vi "test Start Clear.vi"(8 "error in (no error)":errorcluster, 11 "TestCase in":refnum<class "Channel Manager.lvclass">) -> (0 "error out":errorcluster, 3 "TestCase out":refnum<class "Channel Manager.lvclass">)   [LabVIEW 2020, in "Channel Manager.lvclass"]
uses:
  Channel Manager.lvclass
  Hardware API/Channel Status.ctl
  Hardware API/Channel Action.ctl
  <vilib>/addons/_JKI Toolkits/VI Tester/TestCase.llb/TestCase.lvclass
  Hardware API/AIM ARINC 429 Hardware API.lvlib
  C:/Program Files (x86)/National Instruments/LabVIEW 2020/vi.lib/addons/_JKI Toolkits/VI Tester/TestCase.llb/TestCase.lvclass
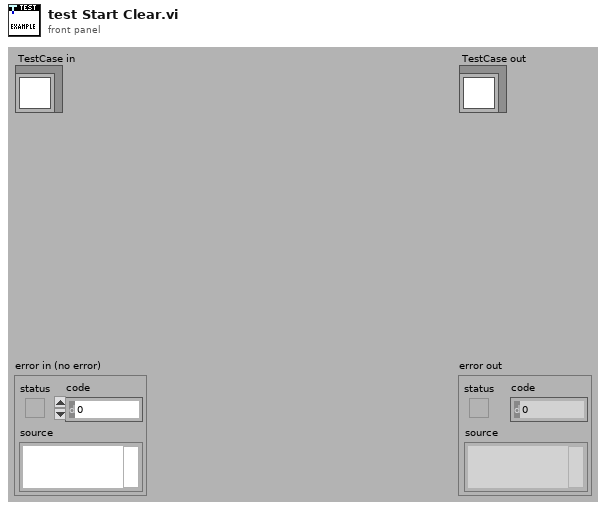
[diagram p1: front panel]
types:
  T1 = typedef "AIM ARINC 429 Hardware API.lvlib/Channel Status.ctl" = enum16{"Uninitialized", "Idle", "Active"}
  T2 = typedef "AIM ARINC 429 Hardware API.lvlib/Channel Action.ctl" = enum16{"Get Info", "Initialize", "Start", "Clear"}
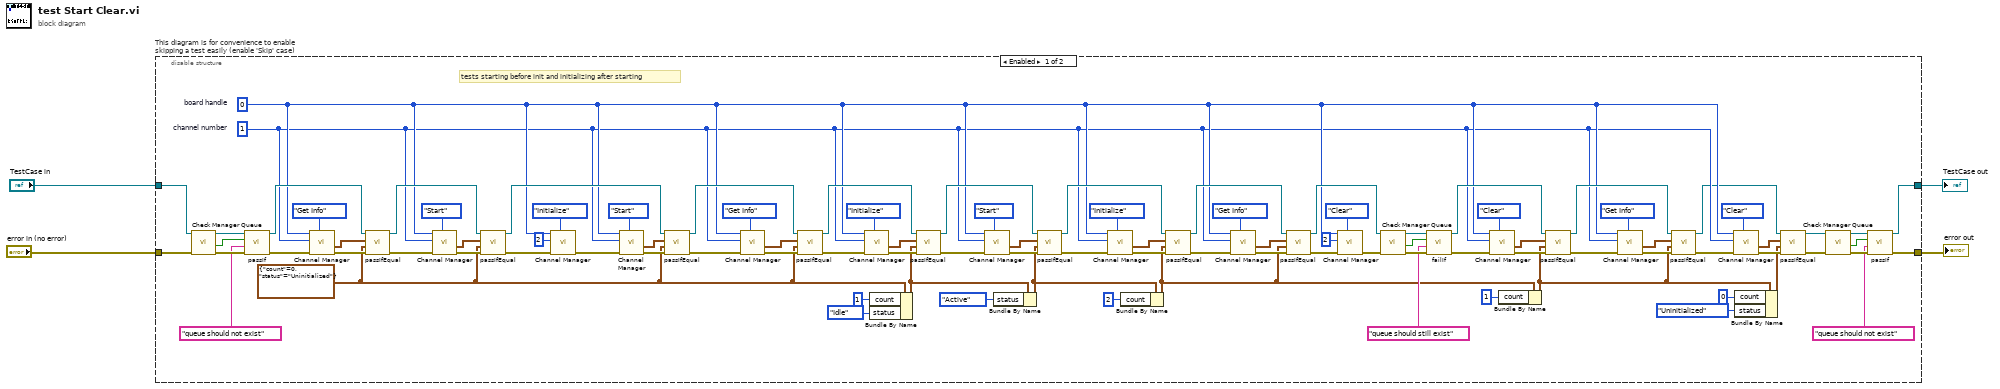
[diagram p0: block diagram]
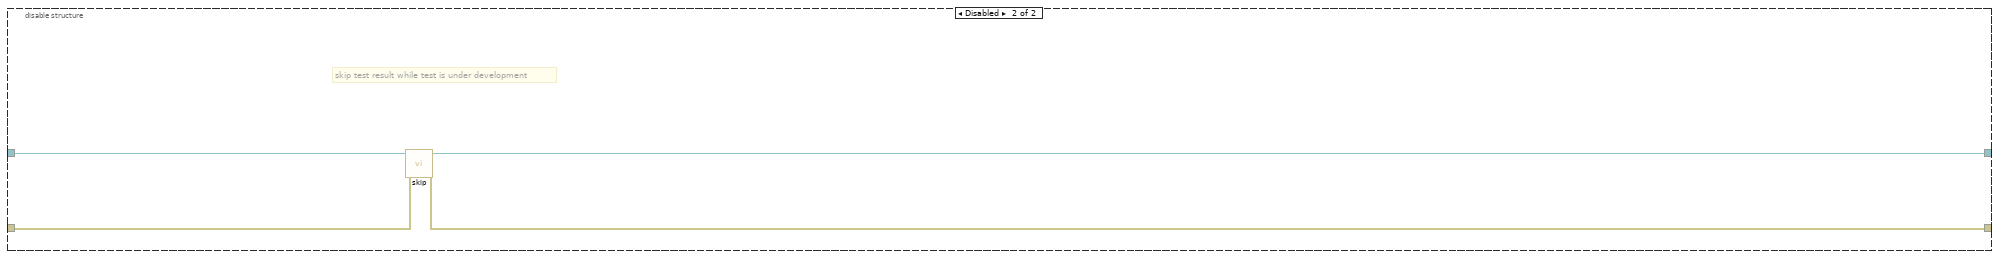
[diagram p2: hidden frame]
diagram:
  n1 = disable-structure "This diagram is for convenience to enable skipping a test easily (enable 'Skip' case)" shown="Enabled" {
    disable-tunnel: "TestCase in" -> [w99 w104]
    disable-tunnel: [w8 w102] -> w1
    disable-tunnel: [w9 w103] -> w3
    disable-tunnel: "error in (no error)" -> [w100 w101]
    frame Enabled {
      w66 = cluster{"count":u32, "status":T1} {"count"=0, "status"=enum."Uninitialized"} ("channel info")
      w20 = u8 1  # channel number
      w21 = u8 0  # board handle
      # "tests starting before init and initializing after starting"
      n2 = call "Check Manager Queue.vi"("error in (no error)"=w100, "Channel Manager in"=w99) -> ("error out"=w98:errorcluster, "queue ref invalid"=w96:bool, "Channel Manager out"=w97:refnum<class "Channel Manager.lvclass">)  [unwired: 7 in]
      n3 = call-dynamic "passIf.vi"("error in (no error)"=w98, "message (\"\")"="queue should not exist" ("message (\"\")"), "pass"=w96, "TestCase in"=w97) -> ("error out"=w94:errorcluster, "TestCase out"=w91:refnum<class "Channel Manager.lvclass">)  [unwired: 6 in]
      n4 = call "Channel Manager.vi"("action"=Channel_Action."Get Info", "error in"=w94, "channel number"=w20, "board handle"=w21) -> ("error out"=w92:errorcluster, "channel info"=w90:cluster{"count":u32, "status":T1})  [unwired: 4 in, 2 out]
      n5 = call-dynamic "passIfEqual.vi"("error in (no error)"=w92, "y"=w66, "x"=w90, "TestCase in"=w91) -> ("error out"=w88:errorcluster, "TestCase out"=w85:refnum<class "Channel Manager.lvclass">)  [unwired: 6 in]
      n6 = call "Channel Manager.vi"("action"=Channel_Action."Start", "error in"=w88, "channel number"=w20, "board handle"=w21) -> ("error out"=w87:errorcluster, "channel info"=w86:cluster{"count":u32, "status":T1})  [unwired: 4 in, 2 out]
      n7 = call-dynamic "passIfEqual.vi"("error in (no error)"=w87, "y"=w66, "x"=w86, "TestCase in"=w85) -> ("error out"=w83:errorcluster, "TestCase out"=w78:refnum<class "Channel Manager.lvclass">)  [unwired: 6 in]
      n8 = call "Channel Manager.vi"("action"=Channel_Action."Initialize", "error in"=w83, "channel number"=u8 2, "board handle"=w21) -> ("error out"=w80:errorcluster)  [unwired: 4 in, 3 out]
      n9 = call "Channel Manager.vi"("action"=Channel_Action."Start", "error in"=w80, "channel number"=w20, "board handle"=w21) -> ("error out"=w79:errorcluster, "channel info"=w77:cluster{"count":u32, "status":T1})  [unwired: 4 in, 2 out]
      n10 = call-dynamic "passIfEqual.vi"("error in (no error)"=w79, "y"=w66, "x"=w77, "TestCase in"=w78) -> ("error out"=w75:errorcluster, "TestCase out"=w74:refnum<class "Channel Manager.lvclass">)  [unwired: 6 in]
      n11 = call "Channel Manager.vi"("action"=Channel_Action."Get Info", "error in"=w75, "channel number"=w20, "board handle"=w21) -> ("error out"=w73:errorcluster, "channel info"=w72:cluster{"count":u32, "status":T1})  [unwired: 4 in, 2 out]
      n12 = call-dynamic "passIfEqual.vi"("error in (no error)"=w73, "y"=w66, "x"=w72, "TestCase in"=w74) -> ("error out"=w70:errorcluster, "TestCase out"=w68:refnum<class "Channel Manager.lvclass">)  [unwired: 6 in]
      n13 = call "Channel Manager.vi"("action"=Channel_Action."Initialize", "error in"=w70, "channel number"=w20, "board handle"=w21) -> ("error out"=w69:errorcluster, "channel info"=w67:cluster{"count":u32, "status":T1})  [unwired: 4 in, 2 out]
      n14 = Bundle By Name(cluster=w66, "count"=u32 1, "status"=Channel_Status."Idle") -> (w58:cluster{"count":u32, "status":T1})
      n15 = call-dynamic "passIfEqual.vi"("error in (no error)"=w69, "y"=w58, "x"=w67, "TestCase in"=w68) -> ("error out"=w62:errorcluster, "TestCase out"=w60:refnum<class "Channel Manager.lvclass">)  [unwired: 6 in]
      n16 = call "Channel Manager.vi"("action"=Channel_Action."Start", "error in"=w62, "channel number"=w20, "board handle"=w21) -> ("error out"=w61:errorcluster, "channel info"=w59:cluster{"count":u32, "status":T1})  [unwired: 4 in, 2 out]
      n17 = Bundle By Name(cluster=w58, "status"=Channel_Status."Active") -> (w50:cluster{"count":u32, "status":T1})
      n18 = call-dynamic "passIfEqual.vi"("error in (no error)"=w61, "y"=w50, "x"=w59, "TestCase in"=w60) -> ("error out"=w55:errorcluster, "TestCase out"=w53:refnum<class "Channel Manager.lvclass">)  [unwired: 6 in]
      n19 = call "Channel Manager.vi"("action"=Channel_Action."Initialize", "error in"=w55, "channel number"=w20, "board handle"=w21) -> ("error out"=w54:errorcluster, "channel info"=w52:cluster{"count":u32, "status":T1})  [unwired: 4 in, 2 out]
      n20 = Bundle By Name(cluster=w50, "count"=u32 2) -> (w30:cluster{"count":u32, "status":T1})
      n21 = call-dynamic "passIfEqual.vi"("error in (no error)"=w54, "y"=w30, "x"=w52, "TestCase in"=w53) -> ("error out"=w48:errorcluster, "TestCase out"=w41:refnum<class "Channel Manager.lvclass">)  [unwired: 6 in]
      n22 = call "Channel Manager.vi"("action"=Channel_Action."Get Info", "error in"=w48, "channel number"=w20, "board handle"=w21) -> ("error out"=w47:errorcluster, "channel info"=w46:cluster{"count":u32, "status":T1})  [unwired: 4 in, 2 out]
      n23 = call-dynamic "passIfEqual.vi"("error in (no error)"=w47, "y"=w30, "x"=w46, "TestCase in"=w41) -> ("error out"=w44:errorcluster, "TestCase out"=w34:refnum<class "Channel Manager.lvclass">)  [unwired: 6 in]
      n24 = call "Channel Manager.vi"("action"=Channel_Action."Clear", "error in"=w44, "channel number"=u8 2, "board handle"=w21) -> ("error out"=w42:errorcluster)  [unwired: 4 in, 3 out]
      n25 = call "Check Manager Queue.vi"("error in (no error)"=w42, "Channel Manager in"=w34) -> ("error out"=w40:errorcluster, "queue ref invalid"=w38:bool, "Channel Manager out"=w39:refnum<class "Channel Manager.lvclass">)  [unwired: 7 in]
      n26 = call-dynamic "failIf.vi"("error in (no error)"=w40, "message (\"\")"="queue should still exist" ("message (\"\")"), "fail"=w38, "TestCase in"=w39) -> ("error out"=w35:errorcluster, "TestCase out"=w32:refnum<class "Channel Manager.lvclass">)  [unwired: 6 in]
      n27 = call "Channel Manager.vi"("action"=Channel_Action."Clear", "error in"=w35, "channel number"=w20, "board handle"=w21) -> ("error out"=w33:errorcluster, "channel info"=w31:cluster{"count":u32, "status":T1})  [unwired: 4 in, 2 out]
      n28 = Bundle By Name(cluster=w30, "count"=u32 1) -> (w18:cluster{"count":u32, "status":T1})
      n29 = call-dynamic "passIfEqual.vi"("error in (no error)"=w33, "y"=w18, "x"=w31, "TestCase in"=w32) -> ("error out"=w27:errorcluster, "TestCase out"=w25:refnum<class "Channel Manager.lvclass">)  [unwired: 6 in]
      n30 = call "Channel Manager.vi"("action"=Channel_Action."Get Info", "error in"=w27, "channel number"=w20, "board handle"=w21) -> ("error out"=w26:errorcluster, "channel info"=w24:cluster{"count":u32, "status":T1})  [unwired: 4 in, 2 out]
      n31 = call-dynamic "passIfEqual.vi"("error in (no error)"=w26, "y"=w18, "x"=w24, "TestCase in"=w25) -> ("error out"=w22:errorcluster, "TestCase out"=w15:refnum<class "Channel Manager.lvclass">)  [unwired: 6 in]
      n32 = call "Channel Manager.vi"("action"=Channel_Action."Clear", "error in"=w22, "channel number"=w20, "board handle"=w21) -> ("error out"=w16:errorcluster, "channel info"=w14:cluster{"count":u32, "status":T1})  [unwired: 4 in, 2 out]
      n33 = Bundle By Name(cluster=w18, "count"=u32 0, "status"=Channel_Status."Uninitialized") -> (w13:cluster{"count":u32, "status":T1})
      n34 = call-dynamic "passIfEqual.vi"("error in (no error)"=w16, "y"=w13, "x"=w14, "TestCase in"=w15) -> ("error out"=w12:errorcluster, "TestCase out"=w11:refnum<class "Channel Manager.lvclass">)  [unwired: 6 in]
      n35 = call "Check Manager Queue.vi"("error in (no error)"=w12, "Channel Manager in"=w11) -> ("error out"=w10:errorcluster, "queue ref invalid"=w6:bool, "Channel Manager out"=w7:refnum<class "Channel Manager.lvclass">)  [unwired: 7 in]
      n36 = call-dynamic "passIf.vi"("error in (no error)"=w10, "message (\"\")"="queue should not exist" ("message (\"\")"), "pass"=w6, "TestCase in"=w7) -> ("error out"=w9:errorcluster, "TestCase out"=w8:refnum<class "Channel Manager.lvclass">)  [unwired: 6 in]
    }
    frame Disabled {
      # "skip test result while test is under development"
      n37 = call <vilib>:"skip.vi"("error in (no error)"=w101, "TestCase in"=w104) -> ("error out"=w103:errorcluster, "TestCase out"=w102:refnum<class "Channel Manager.lvclass">)  [unwired: 8 in]
    }
  }
  "error out" <- w3
  "TestCase out" <- w1
